vi "Read Full Excel Sheet.vi"(8 "Error In":errorcluster, 11 "Excel._Worksheet":refnum<k7>) -> (0 "Error Out":errorcluster, 1 "Data":string[][](array[string]), 3 "Reference Out":refnum<k7>)   [LabVIEW 2013]
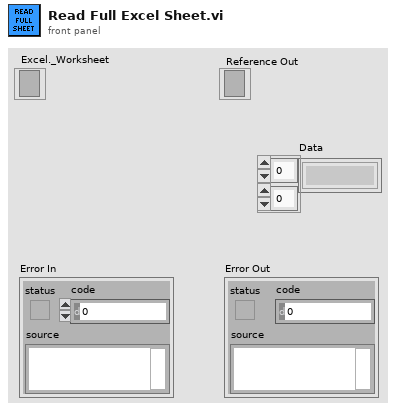
[diagram p1: front panel]
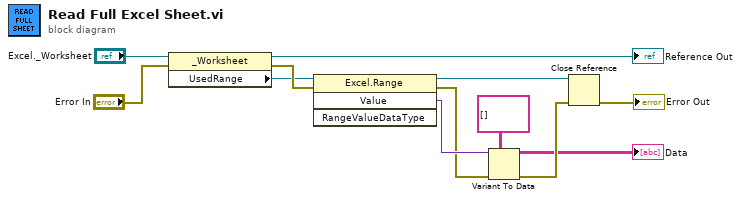
[diagram p0: block diagram]
diagram:
  n1 = property class="_Worksheet"(reference="Excel._Worksheet", error in="Error In") -> (reference out=→"Reference Out":refnum<k7>, error out=w8:errorcluster, "UsedRange"=w5:refnum<k7>)
  n2 = invoke class="Excel.Range" method="Value"(reference=w5, error in=w8) -> (reference out=w7:refnum<k7>, error out=w6:errorcluster, "Value"=w9:variant)  [unwired: 2 in, 1 out]
  n3 = Variant To Data(error in=w6, type=string[][] [], Variant=w9) -> (data=→"Data":string[][], error out=w12:errorcluster)
  n4 = Close Reference(reference=w7, error in (no error)=w12) -> (error out=→"Error Out":errorcluster)
